vi "Query Multi Eval Meas Modulation Absolute Limit Check Results.vi"(0 "VISA resource name":refnum<visa-resource-name>, 5 "Instance (1)":i32=1, 7 "Result Type (Current)":i32(ring) items=["Current"=0, "Average"=1, "Standard Deviation"=3, "Maximum"=4], 11 "error in (no error)":errorcluster) -> (4 "VISA resource name out":refnum<visa-resource-name>, 6 "Reliability":i32, 8 "Out Of Tolerance":i32, 10 "Limit Check Results":dbl[](array[numeric]), 15 "error out":errorcluster)   [LabVIEW 2020, in "Rohde&Schwarz CMP LR WPAN Measurement.lvlib"]
doc: "Returns the absolute limit check single value results.\n\nAttribute:\n-\n\nRemote-control commands:\nCALCulate:WPAN:MEAS<i>:MEValuation:MODulation:ABSolute:CURRent?\nCALCulate:WPAN:MEAS<i>:MEValuation:MODulation:ABSolute:AVERage?\nCALCulate:WPAN:MEAS<i>:MEValuation:MODulation:ABSolute:SDEViation?\nCALCulate:WPAN:MEAS<i>:MEValuation:MODulation:ABSolute:MAXimum?"
uses:
  <instrlib>/Rohde&Schwarz CMP LR WPAN Measurement/Rohde&Schwarz CMP LR WPAN Measurement.lvlib
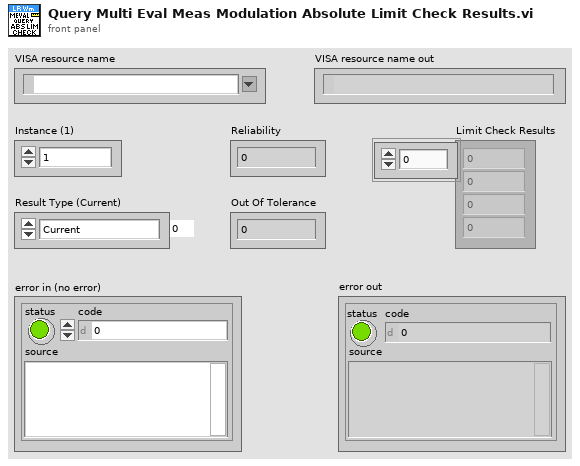
[diagram p1: front panel]
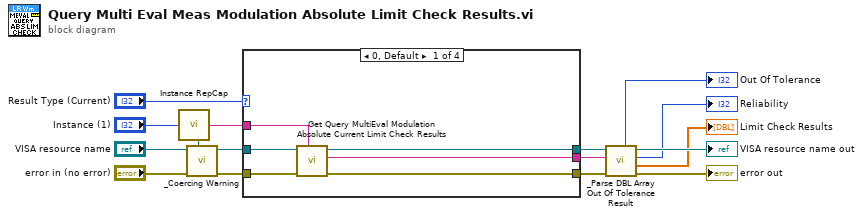
[diagram p0: block diagram]
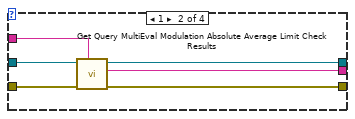
[diagram p2: hidden frame]
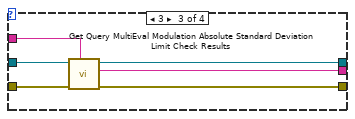
[diagram p3: hidden frame]
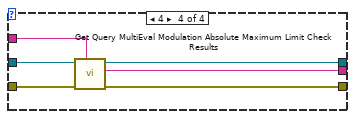
[diagram p4: hidden frame]
diagram:
  n1 = call <instrlib>:"Instance RepCap.vi"("Instance In"="Instance (1)") -> ("In Range?"=w15:bool, "RepCap Identifier Out"=w16:string)  [unwired: 1 in]
  n2 = call <instrlib>:"_Coercing Warning.vi"("In Range?"=w15, "error in (no error)"="error in (no error)", "VISA resource name"="VISA resource name") -> ("error out"=w12:errorcluster, "VISA resource name out"=w11:refnum<visa-resource-name>)  [unwired: 7 in]
  n3 = case shown="0, Default" "Result Type (Current)" {
    tunnel: w16 -> [w22 w28 w34 w38]
    tunnel: w11 -> [w21 w27 w33 w39]
    tunnel: w12 -> [w20 w26 w32 w40]
    tunnel: [w19 w25 w31 w37] -> w9
    tunnel: [w17 w23 w29 w35] -> w3
    tunnel: [w18 w24 w30 w36] -> w2
    frame 0, Default {
      n4 = call "Get Query MultiEval Modulation Absolute Current Limit Check Results"("Repeated Capabilities"=w22, "error in (no error)"=w20, "instrument handle"=w21) -> ("error out"=w17:errorcluster, "Query MultiEval Modulation Absolute Current Limit Check Results"=w18:string, "instrument handle out"=w19:refnum<visa-resource-name>)  [unwired: 6 in]
    }
    frame 1 {
      n5 = call "Get Query MultiEval Modulation Absolute Average Limit Check Results"("Repeated Capabilities"=w28, "error in (no error)"=w26, "instrument handle"=w27) -> ("error out"=w23:errorcluster, "Query MultiEval Modulation Absolute Average Limit Check Results"=w24:string, "instrument handle out"=w25:refnum<visa-resource-name>)  [unwired: 6 in]
    }
    frame 3 {
      n6 = call "Get Query MultiEval Modulation Absolute Standard Deviation Limit Check Results"("Repeated Capabilities"=w34, "error in (no error)"=w32, "instrument handle"=w33) -> ("error out"=w29:errorcluster, "Query MultiEval Modulation Absolute Standard Deviation Limit Check Results"=w30:string, "instrument handle out"=w31:refnum<visa-resource-name>)  [unwired: 6 in]
    }
    frame 4 {
      n7 = call "Get Query MultiEval Modulation Absolute Maximum Limit Check Results"("Repeated Capabilities"=w38, "error in (no error)"=w40, "instrument handle"=w39) -> ("error out"=w35:errorcluster, "Query MultiEval Modulation Absolute Maximum Limit Check Results"=w36:string, "instrument handle out"=w37:refnum<visa-resource-name>)  [unwired: 6 in]
    }
  }
  n8 = call <instrlib>:"_Parse DBL Array Out Of Tolerance Result.vi"("error in (no error)"=w3, "Input String"=w2, "VISA resource name"=w9) -> ("error out"=→"error out":errorcluster, "Results"=→"Limit Check Results":dbl[], "Reliability"=→"Reliability":i32, "VISA resource name out"=→"VISA resource name out":refnum<visa-resource-name>, "Out Of Tolerance"=→"Out Of Tolerance":i32)  [unwired: 4 in]
